vi "Display Color Sequence.vi"(8 "error in (no error)":errorcluster, 11 "GameLogic in":refnum<class "GameLogic.lvclass">) -> (0 "error out":errorcluster, 3 "GameLogic out":refnum<class "GameLogic.lvclass">)   [LabVIEW 2019, in "GameLogic.lvlib" / "GameLogic.lvclass"]
uses:
  GameLogic.lvclass
  GameLogic.lvclass/GameLogic.ctl
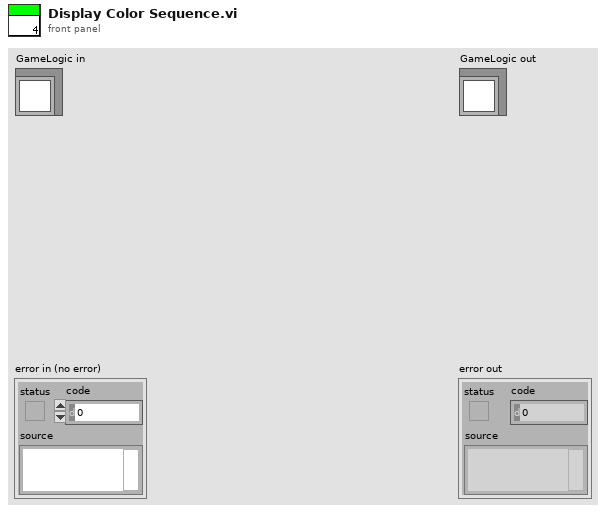
[diagram p1: front panel]
types:
  T1 = cluster{"Blue":bool, "Green":bool, "Red":bool, "Yellow":bool}
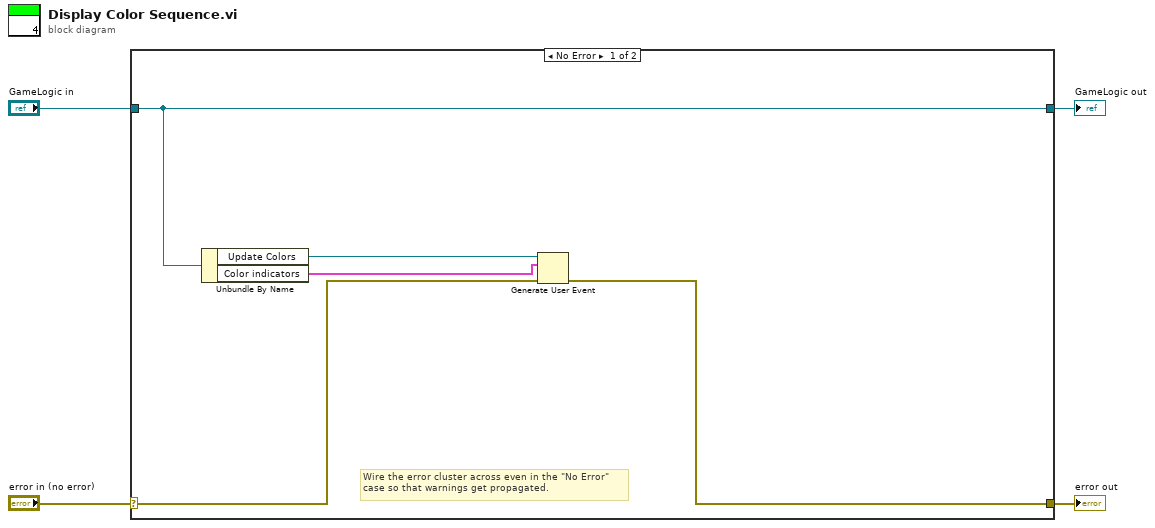
[diagram p0: block diagram]
diagram:
  n1 = case shown="No Error" "error in (no error)" {
    selector: "error in (no error)" -> [w6 w11]
    tunnel: [w5 w11] -> w3
    tunnel: [w9 w10] -> w1
    tunnel: "GameLogic in" -> [w9 w10]
    frame No Error {
      # "Wire the error cluster across even in the \"No Error\"\ncase so that warnings get propagated."
      n2 = Unbundle By Name(w9) -> ("Update Colors"=w8:refnum<user-event>, "Color indicators"=w7:T1)
      n3 = Generate User Event(user event=w8, event data cluster=w7, error in=w6) -> (error out=w5:errorcluster)  [unwired: 1 in, 1 out]
    }
    frame Error {
    }
  }
  "error out" <- w3
  "GameLogic out" <- w1
